vi "Join Sequences.vi"(8 "error in (no error)":errorcluster, 10 "Sequence of SBlocks":refnum<class "Sequence of SBlocks.lvclass">, 11 "Sequence of SBlocks in":refnum<class "Sequence of SBlocks.lvclass">) -> (0 "error out":errorcluster, 3 "Sequence of SBlocks out":refnum<class "Sequence of SBlocks.lvclass">)   [LabVIEW 2020, in "TALOS.lvlib" / "Run Utilities.lvlib" / "Sequence of SBlocks.lvclass"]
uses:
  Sequence of SBlocks.lvclass
  Sequence of SBlocks.lvclass/Sequence of SBlocks.ctl
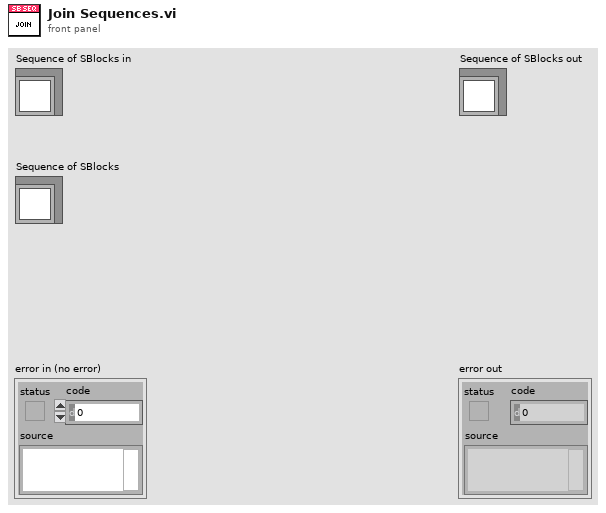
[diagram p1: front panel]
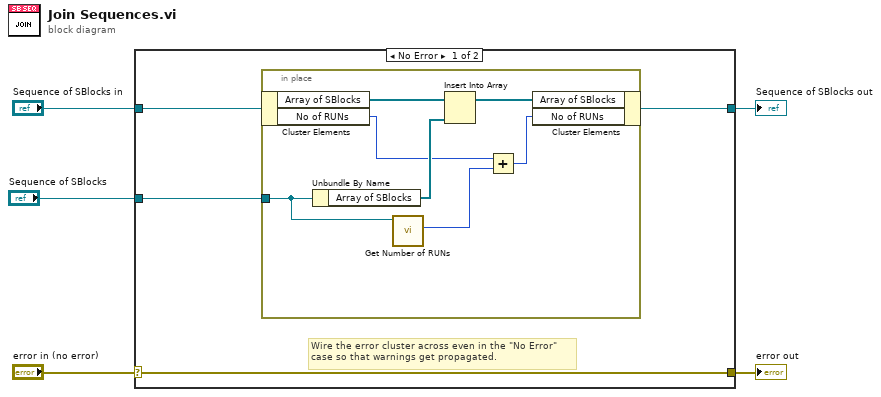
[diagram p0: block diagram]
diagram:
  n1 = case shown="No Error" "error in (no error)" {
    selector: "error in (no error)" -> [w9 w18]
    tunnel: [w9 w18] -> w4
    tunnel: [w6 w17] -> w2
    tunnel: "Sequence of SBlocks in" -> [w8 w17]
    tunnel: "Sequence of SBlocks" -> [w7 _]
    frame No Error {
      # "Wire the error cluster across even in the \"No Error\"\ncase so that warnings get propagated."
      n2 = in-place {
        in-place-border: w7 -> [w13]
        n3 = in-place-cluster #1(w8) -> ("Array of SBlocks"=w16:refnum<class "Schedule Block.lvclass">[], "No of RUNs"=w12:i32)
        n4 = Unbundle By Name(w13) -> ("Array of SBlocks"=w14:refnum<class "Schedule Block.lvclass">[])
        n5 = call-dynamic "Get Number of RUNs.vi"("Sequence of SBlocks in"=w13) -> ("No of RUNs"=w11:i32)  [unwired: 8 in, 2 out]
        n6 = Insert Into Array(array=w16, new element=w14) -> (w15:refnum<class "Schedule Block.lvclass">[])  [unwired: 1 in]
        n7 = Add(x=w12, y=w11) -> (x+y=w10:i32)
        n8 = in-place-cluster #1("Array of SBlocks"=w15, "No of RUNs"=w10) -> (w6:refnum<class "Sequence of SBlocks.lvclass">)
      }
    }
    frame Error {
    }
  }
  "error out" <- w4
  "Sequence of SBlocks out" <- w2
